vi "main.vi"() -> ()   [LabVIEW 2010]
uses:
  <vilib>/Analysis/Matrix/Numeric/Conversions/Array To Matrix - RA2.vi
  <vilib>/Analysis/Matrix/NI_Matrix.lvlib
panel:
  in  "Input":dbl[](array[numeric])
  out "All Possible Codewords":i16[][](array[numeric])
  out "Parities":i16[][](array[numeric])
  out "Msg Comb Boolean":bool[][](array[boolean])
  out "Parties for All Msgs":bool[][](array[boolean])
  out "All Possible combinations for Msg":i16[][](array[numeric])
  out "Generator matrix":dbl[][](array[numeric])
  in  "Parity Matrix":dbl[][](array[numeric])
  in  "k":dbl
  in  "n":dbl
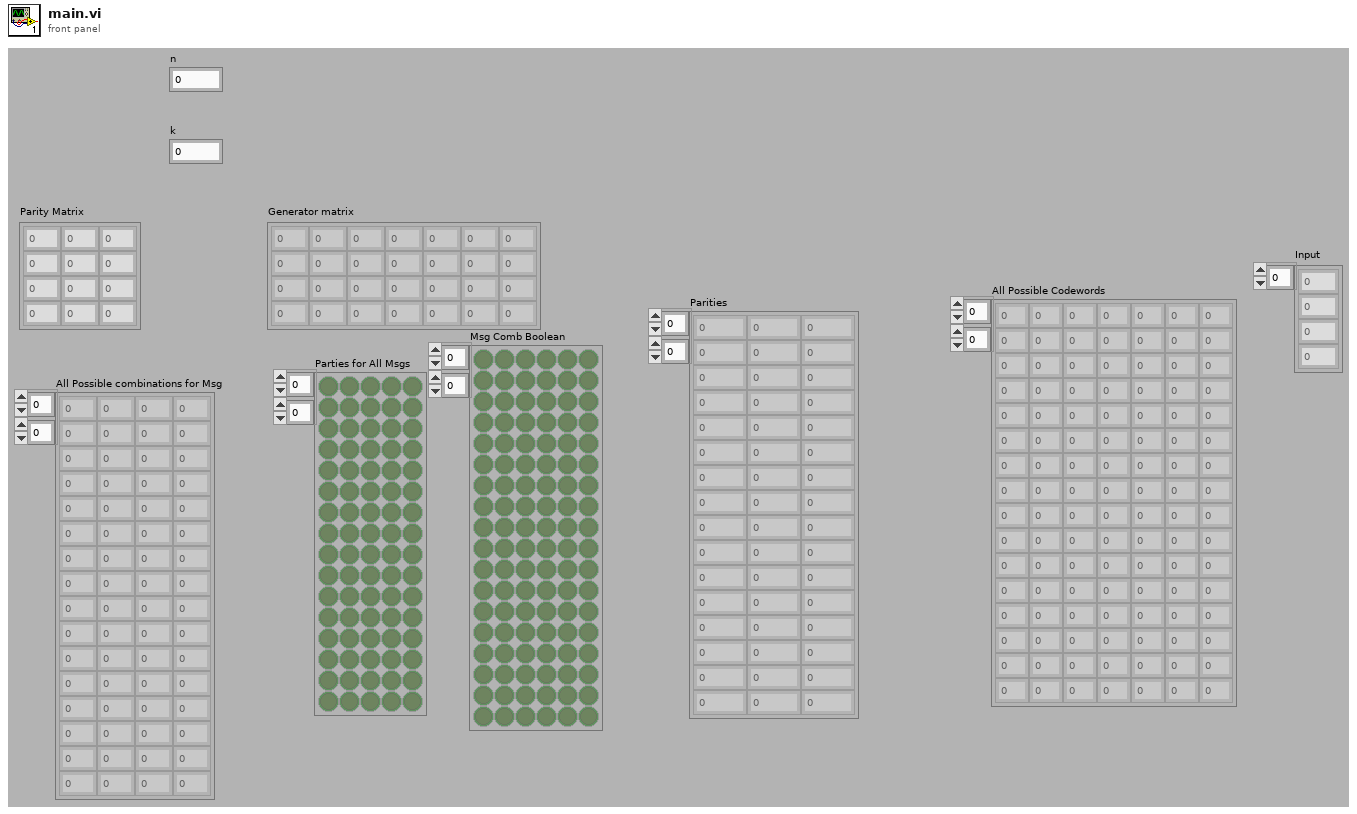
[diagram p1: front panel]
types:
  T1 = typedef "NI_Matrix.lvlib/RealMatrix.ctl" = dbl[][]
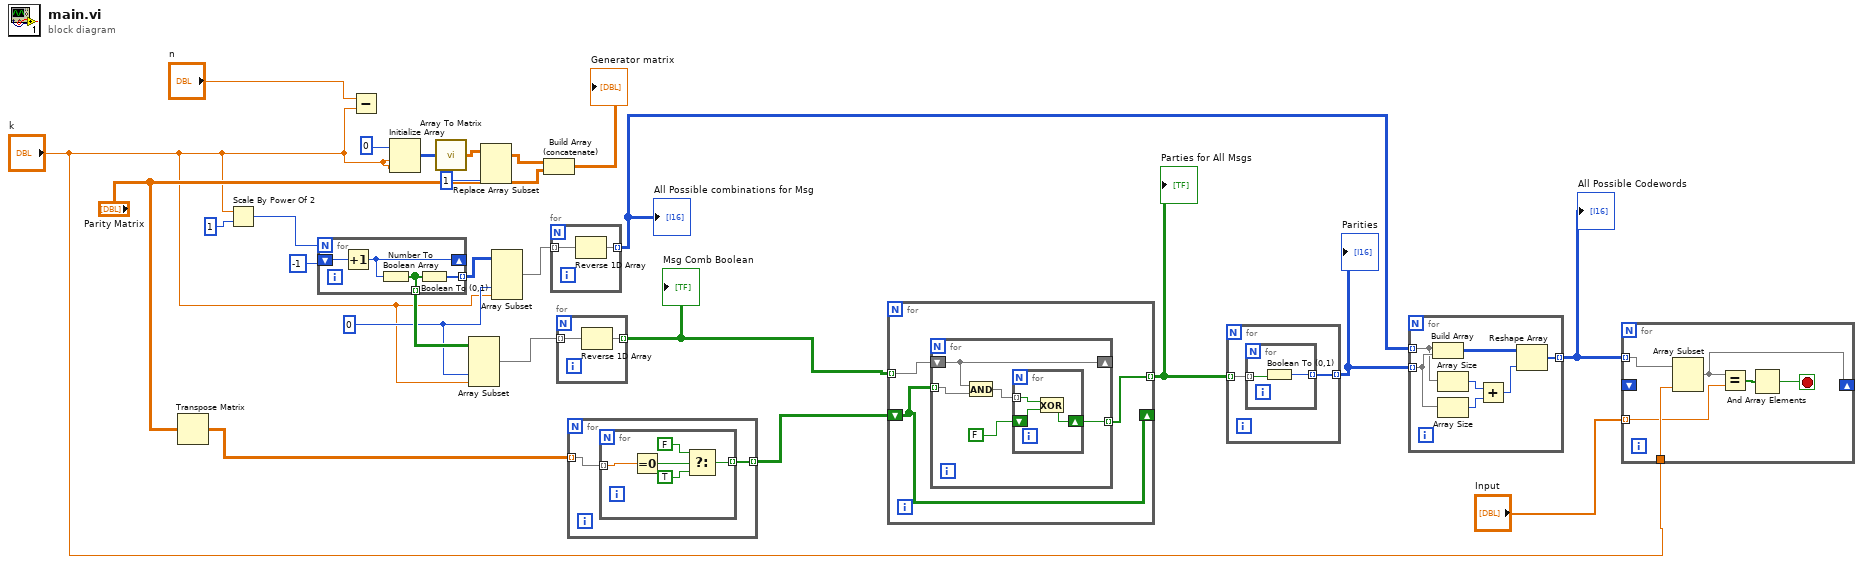
[diagram p0: block diagram]
diagram:
  w9 = 0 ("index")
  n1 = Transpose Matrix(1:"Parity Matrix") -> (0:w14:dbl[][])
  n2 = Scale By Power Of 2(n="k", x=1) -> (x*2^n=w12:i32)
  n3 = for {
    N: w12 -> [_]
    shift-right: [w28] -> _
    shift-left: -1 -> [w29]
    tunnel: [w27] -> w16 mode=indexing
    tunnel: [w26] -> w10 mode=indexing
    n4 = Increment(x=w29) -> (x+1=w28:i32)
    n5 = Number To Boolean Array(number=w28) -> (Boolean array=w26:bool[])
    n6 = Boolean To (0,1)(Boolean=w26) -> (0, 1=w27:i16[])
  }
  n7 = Subtract(x="n", y="k") -> ()  [unwired: 1 out]
  n8 = Initialize Array(0, "k", "k") -> (w22:i32[][])
  n9 = call-poly <vilib>:"Array To Matrix.vi"("Real 2D Array"=w22) -> ("Real Matrix"=w21:T1)
  n10 = Array Subset(array=w10, index (col)=w9, length (col)="k") -> (w8:bool[][])  [unwired: 2 in]
  n11 = Replace Array Subset(array=w21, new element=1) -> (w20:T1)  [unwired: 2 in]
  n12 = Array Subset(array=w16, index (col)=w9, length (col)="k") -> (w7:i16[][])  [unwired: 2 in]
  n13 = Build Array (concatenate)(w20, "Parity Matrix") -> (→"Generator matrix":T1)
  n14 = for {
    tunnel: w7 -> [w31] mode=indexing
    tunnel: [w30] -> w4 mode=indexing
    n15 = Reverse 1D Array(array=w31) -> (reversed array=w30:i16[])
  }
  "All Possible combinations for Msg" <- w4
  n16 = for {
    tunnel: w8 -> [w33] mode=indexing
    tunnel: [w32] -> w11 mode=indexing
    n17 = Reverse 1D Array(array=w33) -> (reversed array=w32:bool[])
  }
  "Msg Comb Boolean" <- w11
  n18 = for {
    tunnel: w14 -> [w35] mode=indexing
    tunnel: [w34] -> w13 mode=indexing
    n19 = for {
      tunnel: w35 -> [w40] mode=indexing
      tunnel: [w36] -> w34 mode=indexing
      n20 = Equal To 0?(x=w40) -> (x = 0?=w39:bool)
      n21 = Select(t=FALSE, s=w39, f=TRUE) -> (s? t:f=w36:bool)
    }
  }
  n22 = for {
    tunnel: w11 -> [w43] mode=indexing
    shift-right: [w42] -> _
    shift-left: w13 -> [w42]
    tunnel: [w41] -> w6 mode=indexing
    n23 = for {
      shift-right: [w48] -> _
      shift-left: w43 -> [w48]
      tunnel: w42 -> [w47] mode=indexing
      tunnel: [w44] -> w41 mode=indexing
      n24 = And(x=w48, y=w47) -> (x .and. y?=w46:bool[])
      n25 = for {
        tunnel: w46 -> [w51] mode=indexing
        shift-right: [w49] -> w44
        shift-left: FALSE -> [w50]
        n26 = Exclusive Or(1:w50, 2:w51) -> (0:w49:bool)
      }
    }
  }
  "Parties for All Msgs" <- w6
  n27 = for {
    tunnel: w6 -> [w53] mode=indexing
    tunnel: [w52] -> w5 mode=indexing
    n28 = for {
      tunnel: w53 -> [w55] mode=indexing
      tunnel: [w54] -> w52 mode=indexing
      n29 = Boolean To (0,1)(Boolean=w55) -> (0, 1=w54:i16)
    }
  }
  "Parities" <- w5
  n30 = for {
    tunnel: w5 -> [w61] mode=indexing
    tunnel: w4 -> [w60] mode=indexing
    tunnel: [w56] -> w3 mode=indexing
    n31 = Build Array(w60, w61) -> (w62:i16[][])
    n32 = Array Size(array=w60) -> (size(s)=w59:i32)
    n33 = Array Size(array=w61) -> (size(s)=w58:i32)
    n34 = Add(x=w59, y=w58) -> (x+y=w57:i32)
    n35 = Reshape Array(w62, w57) -> (w56:i16[])
  }
  "All Possible Codewords" <- w3
  n36 = for {
    tunnel: w3 -> [w67] mode=indexing
    tunnel: "Input" -> [w66] mode=indexing
    tunnel: "k" -> [w68]
    shift-right: [w63] -> _
    shift-left: _ -> [_]
    stop <- w64 stop-if-true
    n37 = Array Subset(array=w67, length=w68) -> (w63:i16[])  [unwired: 1 in]
    n38 = Equal?(x=w63, y=w66) -> (x = y?=w65:bool[])
    n39 = And Array Elements(Boolean array=w65) -> (logical AND=w64:bool)
  }
